vi "Get Is Turned ON.vi"(8 "error in (no error)":errorcluster, 11 "Lamp in":refnum<class "Lamp.lvclass">) -> (0 "error out":errorcluster, 2 "Is Turned ON?":bool, 3 "Lamp out":refnum<class "Lamp.lvclass">)   [LabVIEW 2018, in "Lamp.lvclass"]
uses:
  Lamp.lvclass
  Lamp.lvclass/Lamp.ctl
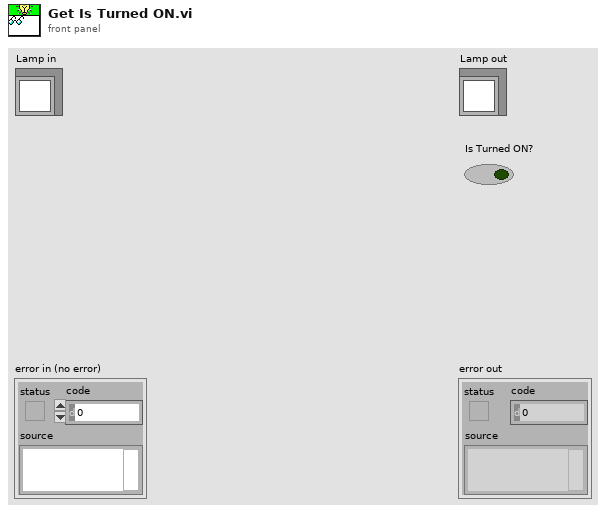
[diagram p1: front panel]
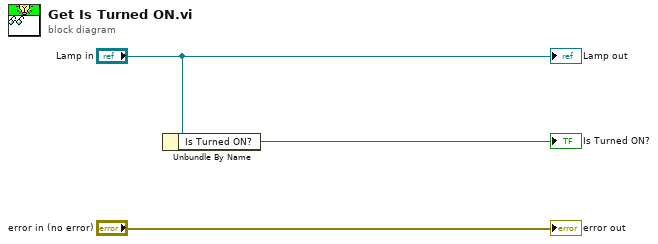
[diagram p0: block diagram]
diagram:
  n1 = Unbundle By Name("Lamp in") -> ("Is Turned ON?"=→"Is Turned ON?":bool)
  "error out" <- "error in (no error)"
  "Lamp out" <- "Lamp in"
